vi "Dashboard Main.vi"() -> ()   [LabVIEW 2012]
uses:
  <vilib>/Rock Robotics/WPI/Solenoid/WPI_SolenoidValue.ctl
  <vilib>/event_ctls.llb/eventvkey.ctl
  <vilib>/Utility/config.llb/Read Key (String).vi
  <vilib>/Utility/config.llb/Read Key (I32).vi
  <vilib>/Utility/config.llb/Write Key (String).vi
  <vilib>/Utility/config.llb/Write Key (I32).vi
  <vilib>/Utility/config.llb/NI_LVConfig.lvlib
panel:
  in  "Run 2":bool
  in  "Run":bool
  in  "Far Speed":dbl=3850.0
  in  "Tower Speed":dbl=2500.0
  out "Camera Image 2":T1(plugin-control)
  in  "Time Delay":dbl
  out "Error":dbl(graph)
  in  "Listbox":i32(listbox)
  out "Shooter Angle":T2
  out "Climb Retical":bool
  out "Primary":T3 {"Slide" scale=-1.0..1.0; "Trigger" scale=-1.0..1.0}
  in  "stop? (T)":bool
  out "RPM":dbl(slide) scale=0.0..5000.0
  out "Right":dbl(slide) scale=-1.0..1.0
  out "Left":dbl(slide) scale=-1.0..1.0
  out "Battery Value":dbl(slide) scale=0.0..14.0 scale format="%#_2e"
  out "Battery":sgl(graph)
  in  "Camera Settings":T4={"Frate Rate"=30, "Compression"=30, "Size"=1} {"Frate Rate" scale=1.0..30.0; "Size" items=["640x480", "320x240", "160x120"]}
  out "Mode":T5(ring)=enum."Auto Disabled"
  out "Camera IP":string
  out "Robot IP":string
  in  "Dashboard Tab":enum32{"Operation", "Test", "Checklist"}(tab)
  in  "Slider":dbl(slide) scale=0.0..100.0 scale format="%#_3g"
  in  "On/Off":bool caption="Solenoid"
  in  "Test Name":u16(ring) items=["Select the test to run...", "Example Test", "-------------------------------", "List of tests is built in robot code.", "Replace with your own automated tests."]
  in  "Test Tree":string(tree)
  in  "Motor":cluster{"Value":dbl, "Enable":bool} {"Value" scale=-1.0..1.0 scale format="%#_3g"}
  out "Progress":T6 {"Test Progress" scale=0.0..100.0}
  in  "Rev/Fwd":cluster{"Forward":bool, "Reverse":bool}
  in  "Ring":u16(ring) items=["Auto", "Fixed indoor", "Fixed outdoor 1", "Fixed outdoor 2", "Fixed fluorescent 1", "Fixed fluorescent 2", "Hold current"]
  in  "Viewer":enum32{"Camera Image", "Variables"}(tab)
  out "Mbps":dbl format="%#.1g"
  in  "Enable":bool=TRUE
  in  "DB Camera Config":bool
  out "Mbps":bool
  out "fps":dbl format="%#.1g"
  out "Image Error Message":string="Timeout in Camera Communications"
  out "Tree":string(tree)
  # "Drive & Motors"
  # "Robot IP:"
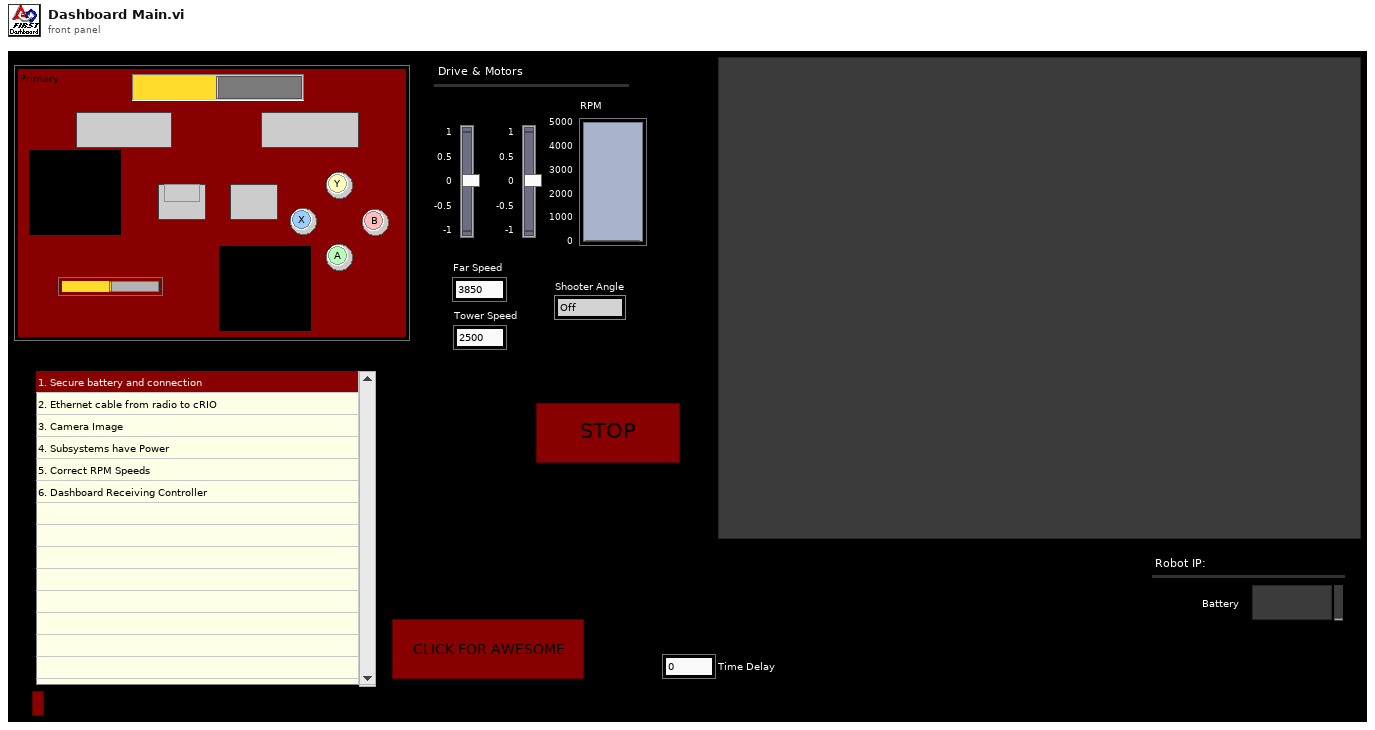
[diagram p1: front panel]
types:
  T1 = typedef "IMAQ Image.ctl" = refnum<image>
  T2 = typedef "WPI_SolenoidValue.ctl" = enum16{"Off", "On", "Forward", "Reverse"}
  T3 = cluster{"Y":bool, "B":bool, "X":bool, "A":bool, "Left Bumper":bool, "Right Bumper":bool, "Joystick 2":cluster{"X":dbl, "Y":dbl}[], "Joystick 3":cluster{"X":dbl, "Y":dbl}[], "Back":bool, "Start":bool, "Trigger":dbl, "Slide":dbl, "Right Thumbstick":bool, "Left Thumbstick":bool}
  T4 = cluster{"Frate Rate":i32, "Compression":i32, "Size":u16}
  T5 = enum8{"Tele-Op Disabled", "Tele-Op Enabled", "Auto Disabled", "Auto Enabled", "Test Disabled", "Test Enabled", ""}
  T6 = cluster{"Test Progress":u8, "Test Progress Text":string}
  T7 = typedef "Image Type" = u32
  T8 = typedef "LVRectTypeDef.ctl" = cluster{"Left":i16, "Top":i16, "Right":i16, "Bottom":i16}
  T9 = cluster{"Joy Stick":cluster{"Primary":cluster{"Buttons":cluster{"A":bool, "B":bool, "X":bool, "Y":bool, "Left Bumper":bool, "Right Bumper":bool, "Back":bool, "Start":bool, "Left Thumbstick":bool, "Right Thumbstick":bool}, "Axes":cluster{"Left Stick X ":dbl, "Left Stick Y":dbl, "Triggers":dbl, "Right Stick X":dbl, "Right Stick Y":dbl, "D-Pad X":dbl}}, "Secondary":cluster{"Buttons":cluster{"A":bool, "B":bool, "X":bool, "Y":bool, "Left Bumper":bool, "Right Bumper":bool, "Back":bool, "Start":bool, "Left Thumbstick":bool, "Right Thumbstick":bool}, "Axes":cluster{"Left Stick X ":dbl, "Left Stick Y":dbl, "Triggers":dbl, "Right Stick X":dbl, "Right Stick Y":dbl, "D-Pad X":dbl}}}, "Shooter":cluster{"RPM Current":dbl, "RPM Set":dbl, "In Range?":bool}, "Arm":cluster{"Arm Current":dbl, "Arm Set":dbl, "At Position?":bool, "Reset Encoder":bool}, "Drive":cluster{"Right":dbl, "Left":dbl}, "Climb State":enum16{"Arm Wait", "Arm Up", "Arm Down", "Arm Attach"}, "Change Retical":bool, "Solenoids":cluster{"Robot Angle":T2, "Shooter Angle":T2, "Arm Lock":T2}, "Shooter Speeds":dbl[]}
  T10 = cluster{"Competition mode":bool, "Robot Link":bool, "Autonomous":bool, "Enabled":bool, "E-Stop":bool, "Simulated":bool, "TestMode":bool, "Docked Window":bool}
  T11 = cluster{"Buttons":cluster{"A":bool, "B":bool, "X":bool, "Y":bool, "Left Bumper":bool, "Right Bumper":bool, "Back":bool, "Start":bool, "Left Thumbstick":bool, "Right Thumbstick":bool}, "Axes":cluster{"Left Stick X ":dbl, "Left Stick Y":dbl, "Triggers":dbl, "Right Stick X":dbl, "Right Stick Y":dbl, "D-Pad X":dbl}}
  T12 = typedef "NI_LVConfig.lvlib/Config Data RefNum.ctl" = refnum<k1>
  T13 = typedef "eventvkey.ctl" = enum16{"ASCII", "Enter", "Return", "Shift", "Ctrl", "Alt", "Cmd", "Opt", "Caps", "NumLock", "Clear", "Break", "Up", "Down", "Left", "Right", "Insert", "Delete", "Home", "End", "PageUp", "PageDown", "Escape", "Help", "Pause", "ScrollLock", "F1", "F2", "F3", "F4", "F5", "F6", "F7", "F8", "F9", "F10", "F11", "F12", "F13", "F14", "F15", "F16", "F17", "F18", "F19", "F20", "F21", "F22", "F23", "F24", "Play", "VolumeUp", "VolumeDown", "Mute", "Two Byte Char"}
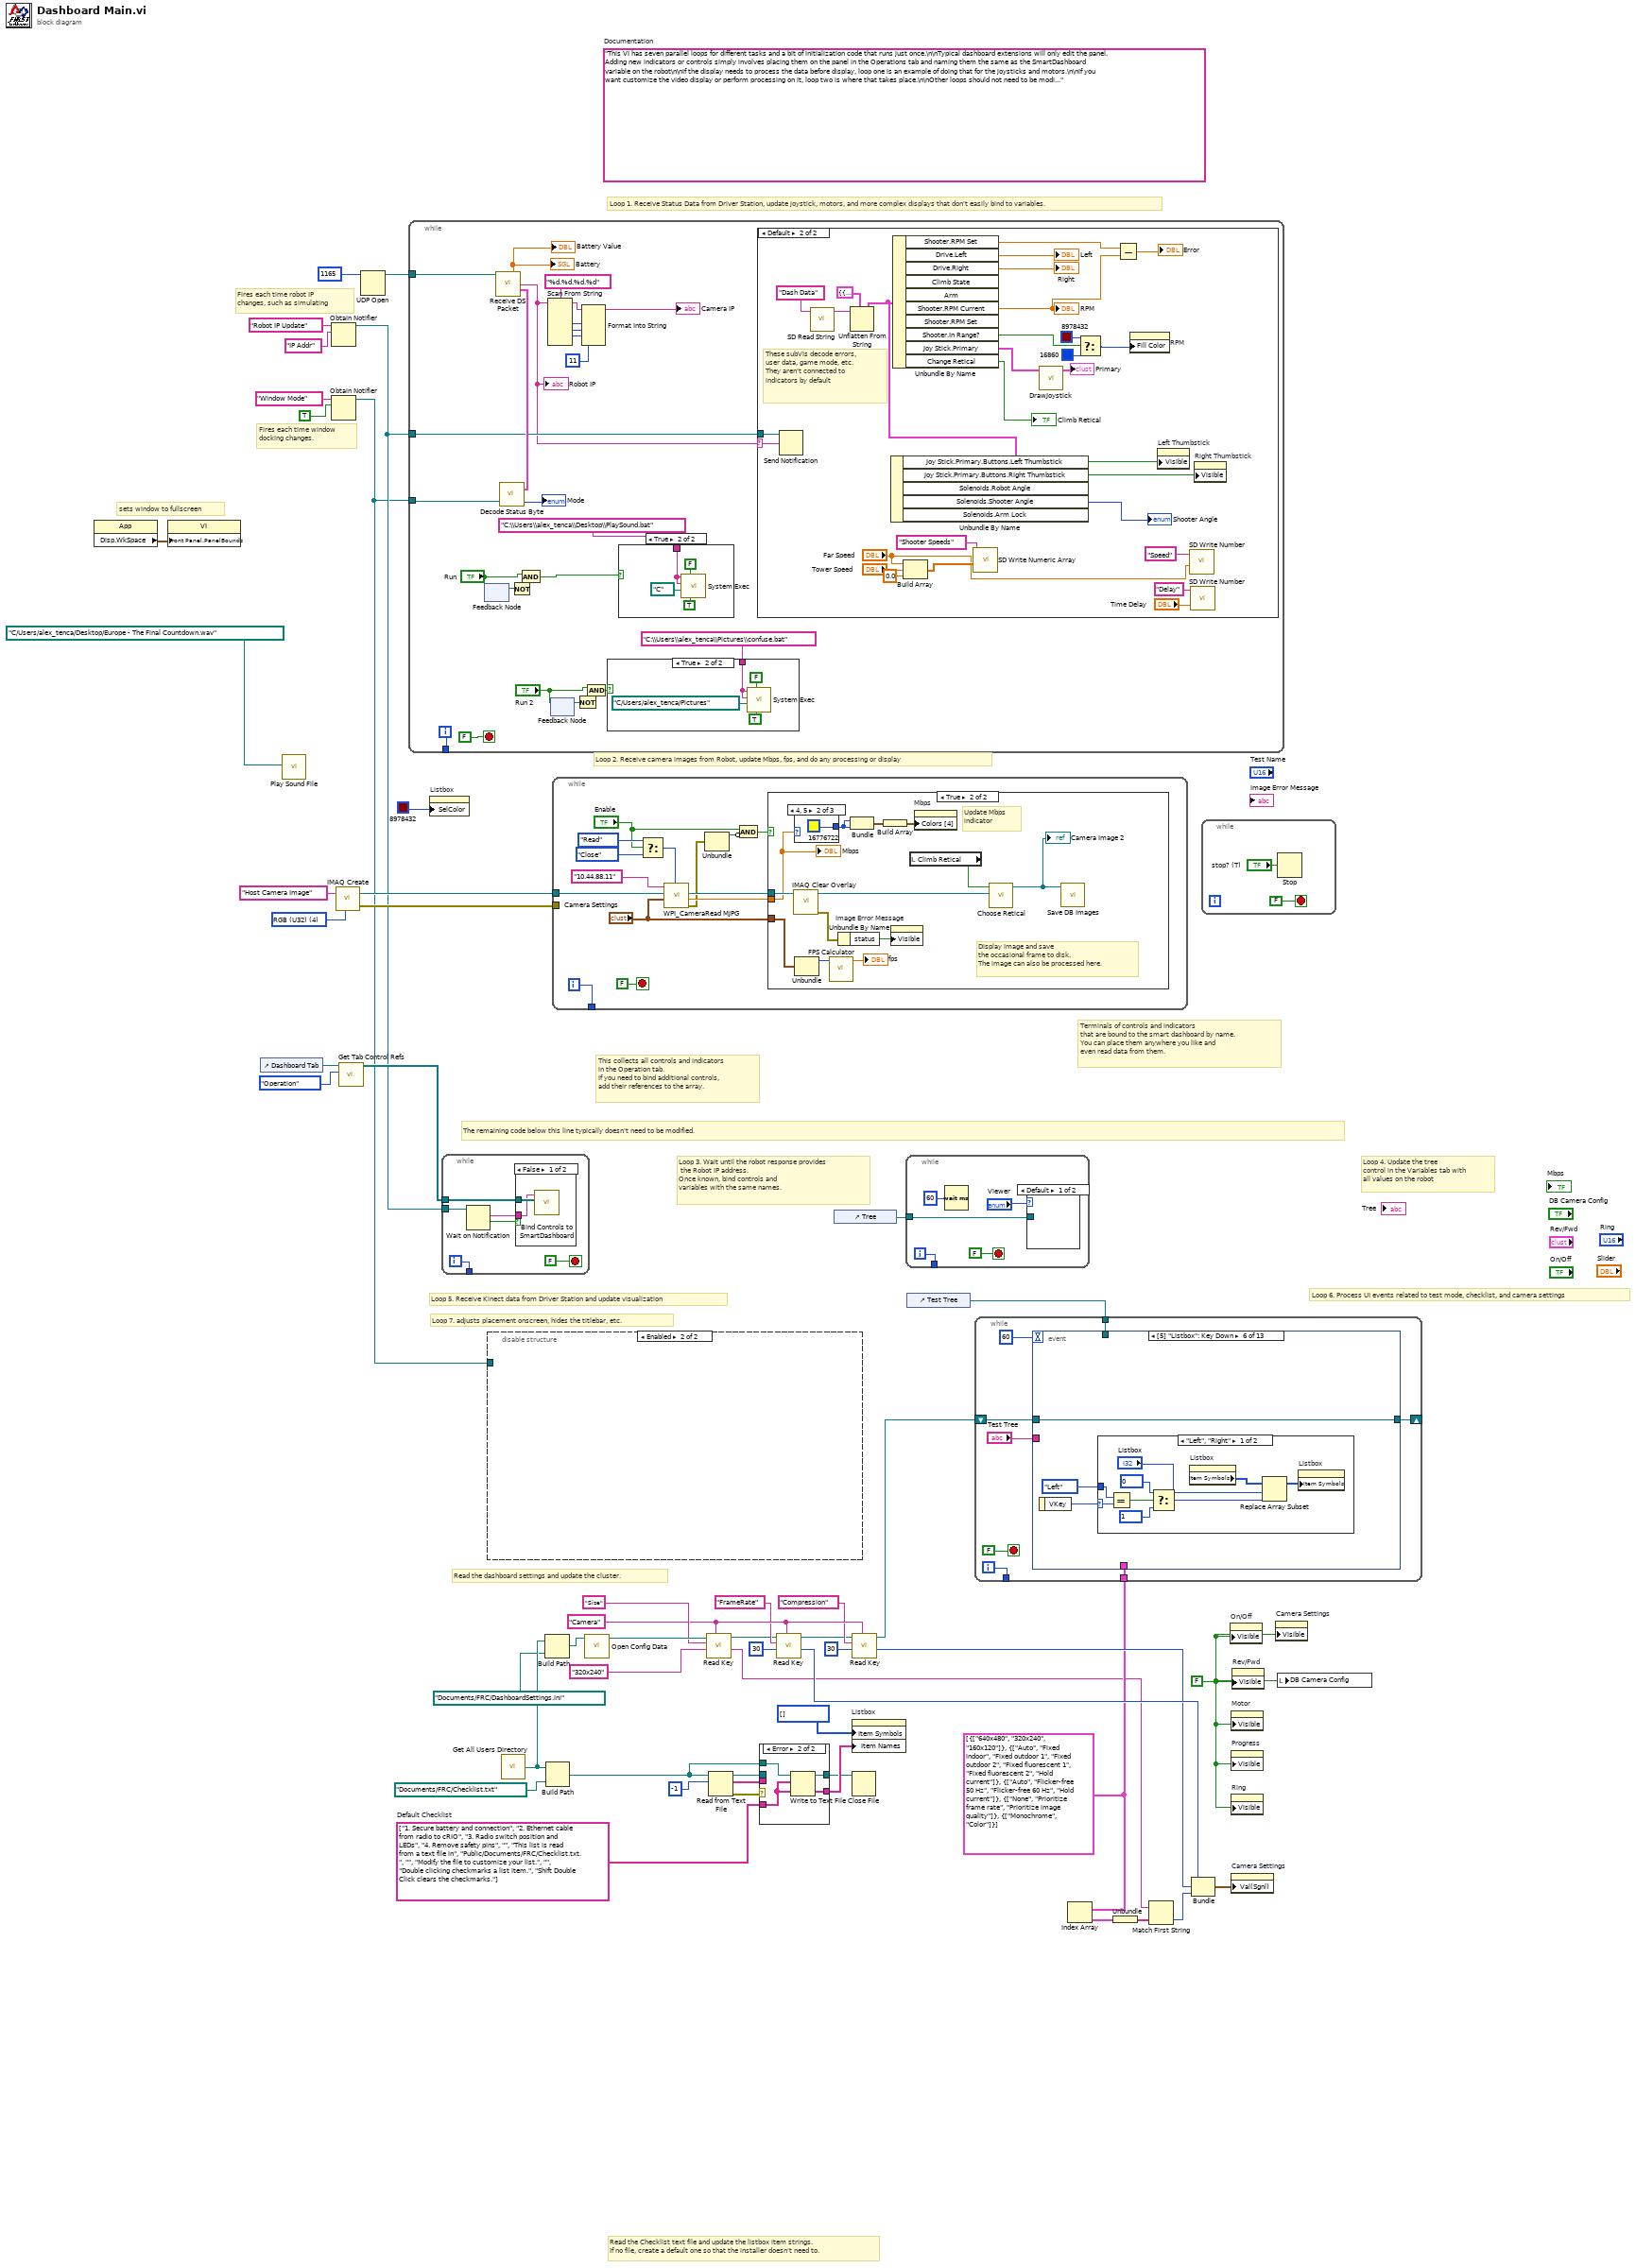
[diagram p0: block diagram]
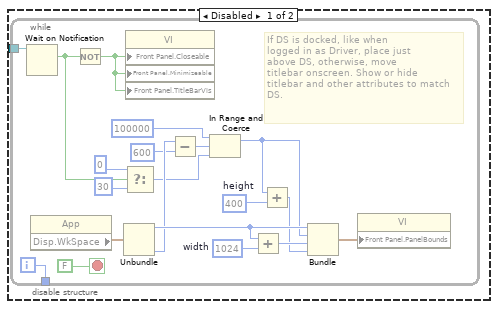
[diagram p2: hidden frame]
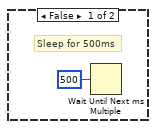
[diagram p4: hidden frame]
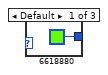
[diagram p5: hidden frame]
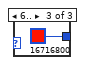
[diagram p6: hidden frame]
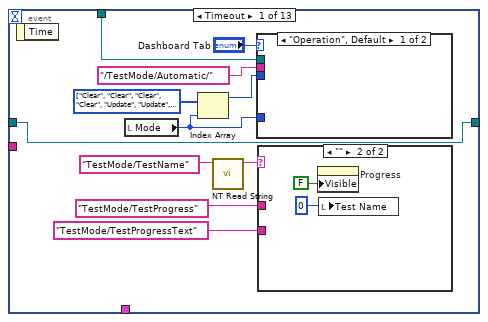
[diagram p8: hidden frame]
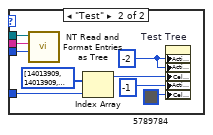
[diagram p9: hidden frame]
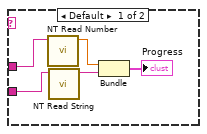
[diagram p10: hidden frame]
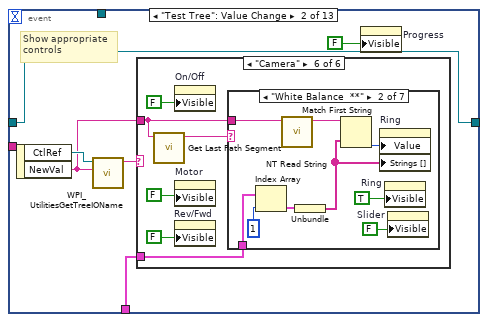
[diagram p11: hidden frame]
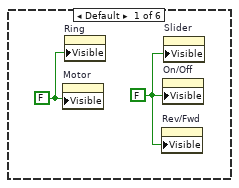
[diagram p12: hidden frame]
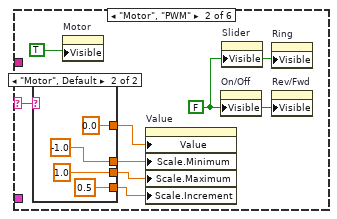
[diagram p13: hidden frame]
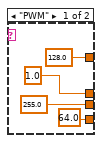
[diagram p14: hidden frame]
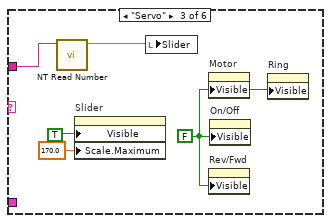
[diagram p15: hidden frame]
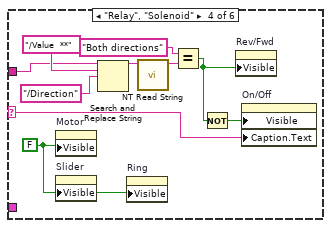
[diagram p16: hidden frame]
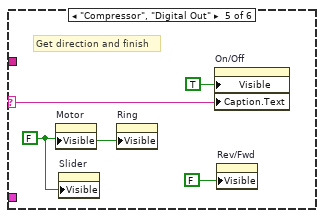
[diagram p17: hidden frame]
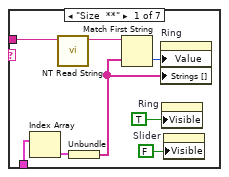
[diagram p18: hidden frame]
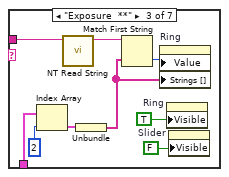
[diagram p19: hidden frame]
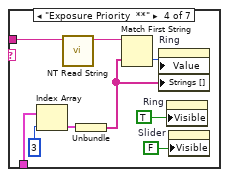
[diagram p20: hidden frame]
diagram:
  w25 = "Camera"
  w17 = cluster{string[]}[] [{["640x480", "320x240", "160x120"]}, {["Auto", "Fixed indoor", "Fixed outdoor 1", "Fixed outdoor 2", "Fixed fluorescent 1", "Fixed fluorescent 2", "Hold current"]}, {["Auto", "Flicker-free 50 Hz", "Flicker-free 60 Hz", "Hold current"]}, {["None", "Prioritize frame rate", "Prioritize image quality"]}, {["Monochrome", "Color"]}]
  w33 = string[] ["1. Secure battery and connection", "2. Ethernet cable from radio to cRIO", "3. Radio switch position and LEDs", "4. Remove safety pins", "", "This list is read from a text file in", "Public/Documents/FRC/Checklist.txt.", "", "Modify the file to customize your list.", "", "Double clicking checkmarks a list item.", "Shift Double Click clears the checkmarks."]  # Default Checklist
  w31 = FALSE ("Visible")
  (unwired) "This VI has seven parallel loops for different tasks and a bit of initialization code that runs just once.\n\nTypical dashboard extensions will only edit the panel. Adding new indicators or controls simply involves placing them on the panel in the Operations tab and naming them the same as the SmartDashboard variable on the robot\n\nIf the display needs to process the data before display, loop one is an example of doing that for the joysticks and motors.\n\nIf you want customize the video display or perform processing on it, loop two is where that takes place.\n\nOther loops should not need to be modified. They are pretty standard, and document the task they perform."  # Documentation
  w51 = T7 4 items=["Grayscale (U8)", "Grayscale (I16)", "Grayscale (SGL)", "Complex (CSG)", "RGB (U32)", "HSL (U32)", "RGB (U64)"] ("Image Type")
  # "sets window to fullscreen"
  # "Fires each time robot IP\nchanges, such as simulating"
  # "Fires each time window\ndocking changes."
  # "Read the Checklist text file and update the listbox item strings.\nIf no file, create a default one so that the installer doesn't need to."
  # "This collects all controls and indicators\nin the Operation tab.\nIf you need to bind additional controls,\nadd their references to the array."
  # "The remaining code below this line typically doesn't need to be modified."
  # "Loop 6. Process UI events related to test mode, checklist, and camera settings"
  # "Read the dashboard settings and update the cluster."
  # "Terminals of controls and indicators\nthat are bound to the smart dashboard by name.\nYou can place them anywhere you like and\neven read data from them."
  # "Loop 4. Update the tree\ncontrol in the Variables tab with\nall values on the robot"
  # "Loop 3. Wait until the robot response provides\n the Robot IP address.\nOnce known, bind controls and\nvariables with the same names."
  # "Loop 5. Receive Kinect data from Driver Station and update visualization"
  # "Loop 7. adjusts placement onscreen, hides the titlebar, etc."
  # "Loop 1. Receive Status Data from Driver Station, update joystick, motors, and more complex displays that don't easily bind to variables."
  # "Loop 2. Receive camera images from Robot, update Mbps, fps, and do any processing or display"
  n1 = property class="App"() -> ("Disp.WkSpace"=w4:T8)  [unwired: 2 in, 2 out]
  n2 = property class="VI"("Front Panel.PanelBounds"=w4) -> ()  [unwired: 2 in, 2 out]
  n3 = control-ref of="Dashboard Tab"() -> (w46:refnum<vi>)
  n4 = call <vilib>:"Play Sound File.vi"("path"=path "C:/Users/alex_tenca/Desktop/Europe - The Final Countdown.wav") -> ()  [unwired: 9 in, 2 out]
  n5 = Obtain Notifier(name (unnamed)="Robot IP Update", notification data type="IP Addr" ("name (unnamed)")) -> (notifier out=w43:refnum<notifier>)  [unwired: 2 in, 2 out]
  n6 = Obtain Notifier(name (unnamed)="Window Mode", notification data type=TRUE) -> (notifier out=w1:refnum<notifier>)  [unwired: 2 in, 2 out]
  n7 = call "IMAQ Create"("Image Name"="Host Camera Image", "Image Type"=w51) -> ("New Image"=w49:T1, "error out"=w48:errorcluster)  [unwired: 2 in, 1 out]
  n8 = call <vilib>:"Get Tab Control Refs.vi"("Page Index"=enum32{"Operation", "Test"}."Operation" ("Dashboard Tab"), "TabControl in"=w46) -> ("ControlsOnPage"=w47:refnum<vi>[])  [unwired: 9 in]
  n9 = UDP Open(11:u16 1165 ("port")) -> (port=w52:refnum<k16>)  [unwired: 2 in, 4 out]
  n10 = while {
    tunnel: w52 -> [w77]
    tunnel: w43 -> [w72]
    tunnel: w1 -> [w75]
    tunnel: [w73] -> _
    i -> [w73]
    stop <- FALSE stop-if-true
    n11 = feedback-in #1("Run") -> ()
    n12 = feedback #1() -> (w62:bool)  [unwired: 1 in]
    n13 = call "Receive DS Packet.vi"("Recv Socket"=w77) -> ("Battery"=→"Battery" →"Battery Value":sgl, "Robot IP Address"=w66:string, "Status"=w78:T10)  [unwired: 1 in, 11 out]
    "Robot IP" <- w66
    n14 = call "Decode Status Byte.vi"("Window Mode Notifier"=w75, "Status"=w78) -> ("Mode"=→"Mode":T5)  [unwired: 1 out]
    n15 = Not(x=w62) -> (.not. x?=w60:bool)
    n16 = And(x="Run", y=w60) -> (x .and. y?=w63:bool)
    n17 = Scan From String(format string="%d.%d.%d.%d", input string=w66) -> (remaining string=w64:string, output 1=w71:i32, output 2=w70:i32, output 3=w69:i32)  [unwired: 2 in, 7 out]
    n18 = feedback #2() -> (w57:bool)  [unwired: 1 in]
    n19 = feedback-in #2("Run 2") -> ()
    n20 = Not(x=w57) -> (.not. x?=w55:bool)
    n21 = Format Into String(initial string=w64, w71, w70, w69, 11 ("IP Suffix:")) -> (resulting string=→"Camera IP":string)  [unwired: 2 in, 1 out]
    n22 = And(x="Run 2", y=w55) -> (x .and. y?=w58:bool)
    n23 = case shown="True" w58 {
      tunnel: "C:\\Users\\alex_tenca\\Pictures\\confuse.bat" ("command line") -> [_ w80]
      frame False {
      }
      frame True {
        n24 = call <vilib>:"System Exec.vi"("run minimized? (F)"=TRUE, "wait until completion? (T)"=FALSE, "working directory"=path "C:/Users/alex_tenca/Pictures", "standard input"=w80, "command line"=w80) -> ()  [unwired: 3 in, 4 out]
      }
    }
    n25 = case shown="True" w63 {
      tunnel: "C:\\Users\\alex_tenca\\Desktop\\PlaySound.bat" ("command line") -> [_ w84]
      frame False {
      }
      frame True {
        n26 = call <vilib>:"System Exec.vi"("run minimized? (F)"=TRUE, "wait until completion? (T)"=FALSE, "working directory"=path "C:/", "standard input"=w84, "command line"=w84) -> ()  [unwired: 3 in, 4 out]
      }
    }
    n27 = case shown="Default" w66 {
      selector: w66 -> [_ w115]
      tunnel: w72 -> [_ w116]
      frame "0.0.0.0" {
        # "Robot not responding, don't poll the variables"
      }
      frame Default {
        # "These subVIs decode errors, user data, game mode, etc.\nThey aren't connected to indicators by default"
        n28 = Send Notification(notification=w115, notifier=w116) -> ()  [unwired: 1 in, 2 out]
        n29 = call <vilib>:"SD Read String.vi"("Name"="Dash Data") -> ("String"=w113:string)  [unwired: 8 in, 2 out]
        n30 = Unflatten From String(type=T9 {"Joy Stick"={"Primary"={"Buttons"={"A"=FALSE, "B"=FALSE, "X"=FALSE, "Y"=FALSE, "Left Bumper"=FALSE, "Right Bumper"=FALSE, "Back"=FALSE, "Start"=FALSE, "Left Thumbstick"=FALSE, "Right Thumbstick"=FALSE}, "Axes"={"Left Stick X "=0.0, "Left Stick Y"=0.0, "Triggers"=-0.0, "Right Stick X"=0.0, "Right Stick Y"=0.0, "D-Pad X"=0.0}}, "Secondary"={"Buttons"={"A"=FALSE, "B"=FALSE, "X"=FALSE, "Y"=FALSE, "Left Bumper"=FALSE, "Right Bumper"=FALSE, "Back"=FALSE, "Start"=FALSE, "Left Thumbstick"=FALSE, "Right Thumbstick"=FALSE}, "Axes"={"Left Stick X "=0.0, "Left Stick Y"=0.0, "Triggers"=0.0, "Right Stick X"=0.0, "Right Stick Y"=0.0, "D-Pad X"=0.0}}}, "Shooter"={"RPM Current"=0.0, "RPM Set"=0.0, "In Range?"=FALSE}, "Arm"={"Arm Current"=0.0, "Arm Set"=0.0, "At Position?"=FALSE, "Reset Encoder"=FALSE}, "Drive"={"Right"=0.0, "Left"=0.0}, "Climb State"=enum."Arm Attach", "Change Retical"=FALSE, "Solenoids"={"Robot Angle"=enum."Off", "Shooter Angle"=enum."Off", "Arm Lock"=enum."Off"}, "Shooter Speeds"=[0.0, 0.0, 0.0]} ("Dash Data"), binary string=w113) -> (value=w109:T9)  [unwired: 3 in, 2 out]
        n31 = Unbundle By Name(w109) -> ("Joy Stick.Primary.Buttons.Left Thumbstick"=w99:bool, "Joy Stick.Primary.Buttons.Right Thumbstick"=w98:bool, "Solenoids.Shooter Angle"=→"Shooter Angle":T2)  [unwired: 2 out]
        n32 = Unbundle By Name(w109) -> ("Shooter.RPM Set"=w107:dbl, "Drive.Left"=→"Left":dbl, "Drive.Right"=→"Right":dbl, "Shooter.RPM Current"=w106:dbl, "Shooter.In Range?"=w104:bool, "Joy Stick.Primary"=w110:T11, "Change Retical"=→"Climb Retical":bool)  [unwired: 3 out]
        "RPM" <- w106
        n33 = Build Array("Far Speed", "Tower Speed", 0.0 ("element")) -> (w92:dbl[])
        n34 = call <vilib>:"SD Write Numeric Array.vi"("Numeric Array"=w92, "Name"="Shooter Speeds") -> ()  [unwired: 8 in, 2 out]
        n35 = call "DrawJoystick.vi"("Joystick"=w110) -> ("DrawJoy"=→"Primary":T3)  [unwired: 10 in]
        n36 = Select(t=u32 8978432 ("Color Box"), s=w104, f=u32 16860 ("Color Box")) -> (s? t:f=w102:u32)
        n37 = Subtract(x=w107, y=w106) -> (x-y=→"Error":dbl)
        n38 = property on="RPM" class="Slide (strict)"("Fill Color"=w102) -> ()  [unwired: 2 in, 2 out]
        n39 = property on="Left Thumbstick" class="Bool (strict)"("Visible"=w99) -> ()  [unwired: 2 in, 2 out]
        n40 = call <vilib>:"SD Write Number.vi"("Numeric"="Far Speed", "Name"="Speed") -> ()  [unwired: 8 in, 2 out]
        n41 = call <vilib>:"SD Write Number.vi"("Numeric"="Time Delay", "Name"="Delay") -> ()  [unwired: 8 in, 2 out]
        n42 = property on="Right Thumbstick" class="Bool (strict)"("Visible"=w98) -> ()  [unwired: 2 in, 2 out]
      }
    }
  }
  n43 = property on="Listbox" class="LstBox (strict)"("SelColor"=u32 8978432 ("Color Box")) -> ()  [unwired: 2 in, 2 out]
  n44 = while {
    tunnel: w47 -> [w122]
    tunnel: w43 -> [w119]
    tunnel: [w117] -> _
    i -> [w117]
    stop <- FALSE stop-if-true
    n45 = Wait on Notification(notifier=w119) -> (notification=w118:string, timed out?=w120:bool)  [unwired: 3 in, 2 out]
    n46 = case shown="False" w120 {
      tunnel: w122 -> [w124 _]
      tunnel: w118 -> [w123 _]
      frame False {
        n47 = call <vilib>:"Bind Controls to SmartDashboard.vi"("Bound Control Refs"=w124, "Server IP Address"=w123) -> ()  [unwired: 10 in]
      }
      frame True {
      }
    }
  }
  n48 = disable-structure shown="Enabled" {
    disable-tunnel: w1 -> [w125 _]
    frame Disabled {
      n49 = while {
        tunnel: w125 -> [w144]
        tunnel: [w142] -> _
        i -> [w142]
        stop <- FALSE stop-if-true
        w134 = 1024  # width
        w137 = 400  # height
        # "If DS is docked, like when\nlogged in as Driver, place just\nabove DS, otherwise, move\ntitlebar onscreen. Show or hide\ntitlebar and other attributes to match\nDS."
        n50 = Wait on Notification(notifier=w144) -> (notification=w129:bool)  [unwired: 3 in, 3 out]
        n51 = property class="App"() -> ("Disp.WkSpace"=w140:T8)  [unwired: 2 in, 2 out]
        n52 = Not(x=w129) -> (.not. x?=w143:bool)
        n53 = Unbundle(w140) -> ("Left"=w138:i16, "Bottom"=w135:i16)  [unwired: 2 out]
        n54 = Select(t=0, s=w129, f=30) -> (s? t:f=w128:i32)
        n55 = property class="VI"("Front Panel.Closeable"=w143, "Front Panel.Minimizeable"=w143, "Front Panel.TitleBarVis"=w143) -> ()  [unwired: 2 in, 2 out]
        n56 = Subtract(x=w135, y=600) -> (x-y=w132:i32)
        n57 = In Range and Coerce(upper limit=100000, x=w132, lower limit=w128) -> (coerced(x)=w126:i32)  [unwired: 1 out]
        n58 = Add(x=w138, y=w134) -> (x+y=w139:i32)
        n59 = Add(x=w126, y=w137) -> (x+y=w136:i32)
        n60 = Bundle("Left"=w138, w126, w139, w136) -> (w141:cluster{"Left":i16, i32, i32, i32})  [unwired: 1 out]
        n61 = property class="VI"("Front Panel.PanelBounds"=w141) -> ()  [unwired: 2 in, 2 out]
      }
    }
    frame Enabled {
    }
  }
  n62 = call "Get All Users Directory.vi"() -> ("All User Path"=w30:path)
  n63 = Build Path(base path=w30, name or relative path=path "Documents/FRC/DashboardSettings.ini") -> (appended path=w29:path)
  n64 = Build Path(base path=w30, name or relative path=path "Documents/FRC/Checklist.txt") -> (appended path=w34:path)
  n65 = while {
    tunnel: w49 -> [w156]
    tunnel: w48 -> [_]
    tunnel: [w158] -> _
    i -> [w158]
    stop <- FALSE stop-if-true
    n66 = Select(t=enum16{"Read", "Reopen", "Close"}."Read" ("Operation"), s="Enable", f=enum16{"Read", "Reopen", "Close"}."Close" ("Operation")) -> (s? t:f=w151:enum16{"Read", "Reopen", "Close"})
    n67 = call <vilib>:"WPI_CameraRead MJPG.vi"("Operation"=w151, "Camera Settings"="Camera Settings", "Image"=w156, "address"="10.44.88.11") -> ("error out"=w150:errorcluster, "Bandwidth (kbps)"=w154:dbl, "Image Out"=w155:T1)  [unwired: 5 in]
    n68 = Unbundle(w150) -> ("status"=w148:bool)  [unwired: 2 out]
    n69 = Compound Arithmetic op=AND("Enable", invert w148) -> (w147:bool)
    n70 = case shown="True" w147 {
      tunnel: "Camera Settings" -> [_ w165]
      tunnel: w155 -> [_ w168]
      tunnel: w154 -> [_ w167]
      frame False {
        # "Sleep for 500ms"
        n71 = Wait Until Next ms Multiple(millisecond multiple=u32 500) -> ()  [unwired: 1 out]
      }
      frame True {
        # "Display image and save\nthe occasional frame to disk.\nThe image can also be processed here."
        # "Update Mbps\nindicator"
        n72 = call "IMAQ Clear Overlay"("Image"=w168) -> ("error out"=w172:errorcluster, "Image Out"=w162:T1)  [unwired: 2 in, 7 out]
        n73 = case shown="4, 5" w167 {
          tunnel: [u32 6618880 ("Color Box") u32 16776722 ("Color Box") u32 16716800 ("Color Box")] -> w169
          frame Default {
          }
          frame 4, 5 {
          }
          frame 6.. {
          }
        }
        n74 = Unbundle(w165) -> ("Frate Rate"=w164:i32)  [unwired: 2 out]
        n75 = call "FPS Calculator.vi"("Average Count"=w164) -> ("fps"=→"fps":dbl)  [unwired: 10 in]
        n76 = Unbundle By Name(w172) -> ("status"=w173:bool)
        n77 = Bundle("Color Box"=w169, "Color Box"=w169) -> (w171:cluster{"Color Box":u32, "Color Box":u32})  [unwired: 1 out]
        n78 = Build Array(w171) -> (w170:cluster{"Color Box":u32, "Color Box":u32}[])
        n79 = property on="Image Error Message" class="Str"("Visible"=w173) -> ()  [unwired: 2 in, 2 out]
        n80 = local read "Climb Retical"() -> (w163:bool)
        n81 = property on="Mbps" class="Bool (strict)"("Colors [4]"=w170) -> ()  [unwired: 2 in, 2 out]
        n82 = call "Choose Retical.vi"("Image In"=w162, "Climb Retical"=w163) -> ("Image Out"=w161:T1)  [unwired: 9 in]
        "Camera Image 2" <- w161
        n83 = call "Save DB Images.vi"("Image"=w161) -> ()  [unwired: 2 in, 1 out]
        "Mbps" <- w167
      }
    }
  }
  n84 = call <vilib>:"Open Config Data.vi"("configuration file path"=w29) -> ("refnum"=w28:T12)  [unwired: 8 in, 2 out]
  n85 = call-poly <vilib>:"Read Key.vi"("section"=w25, "default value"="320x240", "key"="Size", "refnum"=w28) -> ("value"=w15:string, "refnum out"=w10:T12)  [unwired: 2 in, 4 out]
  n86 = Read from Text File(file (use dialog)=w34, count=-1 ("timeout ms (25000)")) -> (refnum out=w12:refnum<file>, text=w35:string[], error out=w36:errorcluster)  [unwired: 2 in, 1 out]
  n87 = case shown="Error" w36 {
    tunnel: w35 -> [w178 _]
    tunnel: [w178 w180] -> w32
    tunnel: w33 -> [_ w180]
    tunnel: w34 -> [_ w181]
    tunnel: [w177 w179] -> w11
    tunnel: w12 -> [w177 _]
    frame No Error {
    }
    frame Error {
      n88 = Write to Text File(file (use dialog)=w181, text=w180) -> (refnum out=w179:refnum<file>)  [unwired: 2 in, 2 out]
    }
  }
  n89 = call-poly <vilib>:"Read Key.vi"("section"=w25, "default value"=30, "key"="FrameRate", "refnum"=w10) -> ("value"=w20:i32, "refnum out"=w9:T12)  [unwired: 1 in, 5 out]
  n90 = control-ref of="Tree"() -> (w6:refnum<vi>)
  n91 = property on="Listbox" class="LstBox (strict)"("Item Symbols"=i32[] [], "Item Names"=w32) -> ()  [unwired: 2 in, 2 out]
  n92 = Close File(refnum=w11) -> ()  [unwired: 1 in, 2 out]
  n93 = call-poly <vilib>:"Read Key.vi"("section"=w25, "default value"=30, "key"="Compression", "refnum"=w9) -> ("value"=w19:i32, "refnum out"=w7:T12)  [unwired: 1 in, 5 out]
  n94 = while {
    tunnel: [w183] -> _
    tunnel: w6 -> [w182]
    i -> [w183]
    stop <- FALSE stop-if-true
    n95 = Wait (ms)(milliseconds to wait=u32 60) -> ()  [unwired: 1 out]
    n96 = case shown="Default" "Viewer" {
      tunnel: w182 -> [_ w187]
      frame Default {
      }
      frame "Variables" {
        n97 = call <vilib>:"NT Read and Format Entries as Tree.vi"("Tree Refnum"=w187) -> ()  [unwired: 9 in, 2 out]
      }
    }
  }
  n98 = control-ref of="Test Tree"() -> (w5:refnum<vi>)
  n99 = while {
    tunnel: w17 -> [w192]
    shift-right: [w191] -> _
    shift-left: w7 -> [w190]
    tunnel: [w189] -> _
    tunnel: w5 -> [w188]
    i -> [w189]
    stop <- FALSE stop-if-true
    n100 = event shown="[5] \"Listbox\": Key Down" {
      selector: _ -> [_ _ _ _ _ _ _ _ _ _ _ _ _]
      dyn-events: _ -> [_ _ _ _ _ _ _ _ _ _ _ _ _]
      timeout: u32 60 ("milliseconds to wait") -> [_ _ _ _ _ _ _ _ _ _ _ _ _]
      tunnel: w188 -> [w202 _ _ _ _ _ _ _ _ _ _ _ _]
      tunnel: "Test Tree" -> [_ _ _ _ _ _ _ _ w396 w404 w406 w410 w418]
      tunnel: w192 -> [_ w224 _ _ _ _ w360 w390 _ _ _ _ _]
      tunnel: [w196 w223 _ w326 w334 w346 w359 w383 w395 w402 w405 w409 w417] -> w191
      tunnel: w190 -> [w196 w223 _ w326 w334 w346 w358 w383 w395 w402 w405 w409 w417]
      event Timeout {
        w201 = enum16{"Update", "Clear"}[] [enum."Clear", enum."Clear", enum."Clear", enum."Clear", enum."Update", enum."Update", enum."Clear"] items=["Update", "Clear"]
        n101 = event-data() -> ()  [unwired: 1 in, 1 out]
        n102 = local read "Mode"() -> (w199:T5)
        n103 = Index Array(array=w201, index=w199) -> (element=w200:enum16{"Update", "Clear"})
        n104 = call <vilib>:"NT Read String.vi"("Name"="TestMode/TestName") -> ("String"=w205:string)  [unwired: 9 in, 1 out]
        n105 = case shown="\"Operation\", Default" "Dashboard Tab" {
          tunnel: w202 -> [_ w215]
          tunnel: "/TestMode/Automatic/" ("Name Pattern") -> [_ w214]
          tunnel: w200 -> [_ w213]
          tunnel: w199 -> [_ w211]
          frame "Operation", Default {
          }
          frame "Test" {
            w210 = -2 ("Active Item:Row Number")
            n106 = call <vilib>:"NT Read and Format Entries as Tree.vi"("Operation"=w213, "Name Pattern"=w214, "Tree Refnum"=w215) -> ()  [unwired: 7 in, 2 out]
            n107 = Index Array(array=u32[] [14013909, 14013909, 14013909, 14013909, 14013909, 16777215, 14013909], index=w211) -> (element=w209:u32)
            n108 = property on="Test Tree" class="Tree (strict)"("Active Item Row Number"=w210, "ActiveColNum"=w210, "CellBG"=w209, "Active Item Row Number"=-1 ("Active Item:Row Number"), "CellBG"=u32 5789784 ("Color Box")) -> ()  [unwired: 2 in, 2 out]
          }
        }
        n109 = case shown="\"\"" w205 {
          tunnel: "TestMode/TestProgress" ("Name") -> [w217 _]
          tunnel: "TestMode/TestProgressText" ("Name") -> [w216 _]
          frame Default {
            n110 = call <vilib>:"NT Read Number.vi"("Name"=w217) -> ("Numeric"=w218:dbl)  [unwired: 9 in, 1 out]
            n111 = call <vilib>:"NT Read String.vi"("Name"=w216) -> ("String"=w219:string)  [unwired: 9 in, 1 out]
            n112 = Bundle("Numeric"=w218, "String"=w219) -> (→"Progress":cluster{"Numeric":dbl, "String":string})  [unwired: 1 in]
          }
          frame "" {
            n113 = property on="Progress" class="Clust (strict)"("Visible"=FALSE) -> ()  [unwired: 2 in, 2 out]
            n114 = local write "Test Name"(u16 0) -> ()
          }
        }
      }
      event "Test Tree": Value Change {
        # "Show appropriate\ncontrols"
        n115 = event-data() -> ("CtlRef"=w227:refnum<vi>, "NewVal"=w225:string)  [unwired: 1 in]
        n116 = call <vilib>:"WPI_UtilitiesGetTreeIOName.vi"("NewVal"=w225, "TreeControl in"=w227) -> ("I/O Name"=w228:string)  [unwired: 9 in]
        n117 = case shown="\"Camera\"" w228 {
          selector: w228 -> [_ w235 _ w253 w262 _]
          tunnel: w225 -> [_ _ w250 w252 _ w269]
          tunnel: w224 -> [_ _ _ _ _ w268]
          frame Default {
            w230 = FALSE ("Visible")
            w229 = FALSE ("Visible")
            n118 = property on="Motor" class="Clust (strict)"("Visible"=w229) -> ()  [unwired: 2 in, 2 out]
            n119 = property on="Ring" class="Ring (strict)"("Visible"=w229) -> ()  [unwired: 2 in, 2 out]
            n120 = property on="Rev/Fwd" class="Clust (strict)"("Visible"=w230) -> ()  [unwired: 2 in, 2 out]
            n121 = property on="On/Off" class="Bool (strict)"("Visible"=w230) -> ()  [unwired: 2 in, 2 out]
            n122 = property on="Slider" class="Slide (strict)"("Visible"=w230) -> ()  [unwired: 2 in, 2 out]
          }
          frame "Motor", "PWM" {
            w236 = FALSE ("Visible")
            n123 = case shown="\"Motor\", Default" w235 {
              tunnel: [1.0 ("Value") -1.0 ("Value")] -> w234
              tunnel: [255.0 ("Value") 1.0 ("Value")] -> w233
              tunnel: [128.0 ("Value") 0.0 ("Value")] -> w232
              tunnel: [64.0 ("Value") 0.5 ("Value")] -> w231
              frame "PWM" {
              }
              frame "Motor", Default {
              }
            }
            n124 = property on="Motor" class="Clust (strict)"("Visible"=TRUE) -> ()  [unwired: 2 in, 2 out]
            n125 = property on="Value" class="Slide (strict)"("Value"=w232, "Scale.Minimum"=w234, "Scale.Maximum"=w233, "Scale.Increment"=w231) -> ()  [unwired: 2 in, 2 out]
            n126 = property on="On/Off" class="Bool (strict)"("Visible"=w236) -> ()  [unwired: 2 in, 2 out]
            n127 = property on="Slider" class="Slide (strict)"("Visible"=w236) -> ()  [unwired: 2 in, 2 out]
            n128 = property on="Ring" class="Ring (strict)"("Visible"=w236) -> ()  [unwired: 2 in, 2 out]
            n129 = property on="Rev/Fwd" class="Clust (strict)"("Visible"=w236) -> ()  [unwired: 2 in, 2 out]
          }
          frame "Servo" {
            w248 = FALSE ("Visible")
            n130 = call <vilib>:"NT Read Number.vi"("Name"=w250) -> ("Numeric"=w249:dbl)  [unwired: 9 in, 1 out]
            n131 = property on="Slider" class="Slide (strict)"("Visible"=TRUE, "Scale.Maximum"=170.0 ("Scale.Range:Maximum")) -> ()  [unwired: 2 in, 2 out]
            n132 = local write "Slider"(w249) -> ()
            n133 = property on="Motor" class="Clust (strict)"("Visible"=w248) -> ()  [unwired: 2 in, 2 out]
            n134 = property on="Rev/Fwd" class="Clust (strict)"("Visible"=w248) -> ()  [unwired: 2 in, 2 out]
            n135 = property on="On/Off" class="Bool (strict)"("Visible"=w248) -> ()  [unwired: 2 in, 2 out]
            n136 = property on="Ring" class="Ring (strict)"("Visible"=w248) -> ()  [unwired: 2 in, 2 out]
          }
          frame "Relay", "Solenoid" {
            w251 = FALSE ("Visible")
            n137 = property on="Motor" class="Clust (strict)"("Visible"=w251) -> ()  [unwired: 2 in, 2 out]
            n138 = property on="Slider" class="Slide (strict)"("Visible"=w251) -> ()  [unwired: 2 in, 2 out]
            n139 = Search and Replace String(input string=w252, search string="/Value  **", replace string="/Direction") -> (result string=w258:string)  [unwired: 5 in, 3 out]
            n140 = property on="Ring" class="Ring (strict)"("Visible"=w251) -> ()  [unwired: 2 in, 2 out]
            n141 = call <vilib>:"NT Read String.vi"("Name"=w258) -> ("String"=w256:string)  [unwired: 9 in, 1 out]
            n142 = Equal?(x="Both directions", y=w256) -> (x = y?=w254:bool)
            n143 = Not(x=w254) -> (.not. x?=w255:bool)
            n144 = property on="Rev/Fwd" class="Clust (strict)"("Visible"=w254) -> ()  [unwired: 2 in, 2 out]
            n145 = property on="On/Off" class="Bool (strict)"("Visible"=w255, "Caption.Text"=w253) -> ()  [unwired: 2 in, 2 out]
          }
          frame "Compressor", "Digital Out" {
            w261 = FALSE ("Visible")
            # "Get direction and finish"
            n146 = property on="Motor" class="Clust (strict)"("Visible"=w261) -> ()  [unwired: 2 in, 2 out]
            n147 = property on="Slider" class="Slide (strict)"("Visible"=w261) -> ()  [unwired: 2 in, 2 out]
            n148 = property on="Ring" class="Ring (strict)"("Visible"=w261) -> ()  [unwired: 2 in, 2 out]
            n149 = property on="On/Off" class="Bool (strict)"("Visible"=TRUE, "Caption.Text"=w262) -> ()  [unwired: 2 in, 2 out]
            n150 = property on="Rev/Fwd" class="Clust (strict)"("Visible"=FALSE) -> ()  [unwired: 2 in, 2 out]
          }
          frame "Camera" {
            n151 = call <vilib>:"Get Last Path Segment.vi"("String in"=w269) -> ("String out"=w270:string)  [unwired: 10 in]
            n152 = property on="On/Off" class="Bool (strict)"("Visible"=FALSE) -> ()  [unwired: 2 in, 2 out]
            n153 = property on="Motor" class="Clust (strict)"("Visible"=FALSE) -> ()  [unwired: 2 in, 2 out]
            n154 = property on="Rev/Fwd" class="Clust (strict)"("Visible"=FALSE) -> ()  [unwired: 2 in, 2 out]
            n155 = case shown="\"White Balance  **\"" w270 {
              tunnel: w269 -> [w276 w285 w294 w303 w312 _ w318]
              tunnel: w268 -> [w274 w282 w291 w300 w309 _ _]
              frame "Size  **" {
                n156 = Index Array(array=w274) -> (element=w273:cluster{string[]})  [unwired: 1 in]
                n157 = call <vilib>:"NT Read String.vi"("Name"=w276) -> ("String"=w275:string)  [unwired: 9 in, 1 out]
                n158 = Unbundle(w273) -> (w271:string[])
                n159 = Match First String(2:w271, 3:w275) -> (0:w272:i32)  [unwired: 1 out]
                n160 = property on="Ring" class="Ring (strict)"("Value"=w272, "Strings []"=w271) -> ()  [unwired: 2 in, 2 out]
                n161 = property on="Ring" class="Ring (strict)"("Visible"=TRUE) -> ()  [unwired: 2 in, 2 out]
                n162 = property on="Slider" class="Slide (strict)"("Visible"=FALSE) -> ()  [unwired: 2 in, 2 out]
              }
              frame "White Balance  **" {
                n163 = Index Array(array=w282, index=1) -> (element=w283:cluster{string[]})
                n164 = call <vilib>:"NT Read String.vi"("Name"=w285) -> ("String"=w284:string)  [unwired: 9 in, 1 out]
                n165 = Unbundle(w283) -> (w280:string[])
                n166 = Match First String(2:w280, 3:w284) -> (0:w279:i32)  [unwired: 1 out]
                n167 = property on="Ring" class="Ring (strict)"("Value"=w279, "Strings []"=w280) -> ()  [unwired: 2 in, 2 out]
                n168 = property on="Ring" class="Ring (strict)"("Visible"=TRUE) -> ()  [unwired: 2 in, 2 out]
                n169 = property on="Slider" class="Slide (strict)"("Visible"=FALSE) -> ()  [unwired: 2 in, 2 out]
              }
              frame "Exposure  **" {
                n170 = Index Array(array=w291, index=2) -> (element=w292:cluster{string[]})
                n171 = call <vilib>:"NT Read String.vi"("Name"=w294) -> ("String"=w293:string)  [unwired: 9 in, 1 out]
                n172 = Unbundle(w292) -> (w288:string[])
                n173 = Match First String(2:w288, 3:w293) -> (0:w289:i32)  [unwired: 1 out]
                n174 = property on="Ring" class="Ring (strict)"("Value"=w289, "Strings []"=w288) -> ()  [unwired: 2 in, 2 out]
                n175 = property on="Ring" class="Ring (strict)"("Visible"=TRUE) -> ()  [unwired: 2 in, 2 out]
                n176 = property on="Slider" class="Slide (strict)"("Visible"=FALSE) -> ()  [unwired: 2 in, 2 out]
              }
              frame "Exposure Priority  **" {
                n177 = Index Array(array=w300, index=3) -> (element=w301:cluster{string[]})
                n178 = call <vilib>:"NT Read String.vi"("Name"=w303) -> ("String"=w302:string)  [unwired: 9 in, 1 out]
                n179 = Unbundle(w301) -> (w297:string[])
                n180 = Match First String(2:w297, 3:w302) -> (0:w298:i32)  [unwired: 1 out]
                n181 = property on="Ring" class="Ring (strict)"("Value"=w298, "Strings []"=w297) -> ()  [unwired: 2 in, 2 out]
                n182 = property on="Ring" class="Ring (strict)"("Visible"=TRUE) -> ()  [unwired: 2 in, 2 out]
                n183 = property on="Slider" class="Slide (strict)"("Visible"=FALSE) -> ()  [unwired: 2 in, 2 out]
              }
              frame "Color Enable  **" {
                n184 = Index Array(array=w309, index=4) -> (element=w310:cluster{string[]})
                n185 = call <vilib>:"NT Read String.vi"("Name"=w312) -> ("String"=w311:string)  [unwired: 9 in, 1 out]
                n186 = Unbundle(w310) -> (w306:string[])
                n187 = Match First String(2:w306, 3:w311) -> (0:w307:i32)  [unwired: 1 out]
                n188 = property on="Ring" class="Ring (strict)"("Value"=w307, "Strings []"=w306) -> ()  [unwired: 2 in, 2 out]
                n189 = property on="Ring" class="Ring (strict)"("Visible"=TRUE) -> ()  [unwired: 2 in, 2 out]
                n190 = property on="Slider" class="Slide (strict)"("Visible"=FALSE) -> ()  [unwired: 2 in, 2 out]
              }
              frame Default {
                n191 = property on="Ring" class="Ring (strict)"("Visible"=FALSE) -> ()  [unwired: 2 in, 2 out]
                n192 = property on="Slider" class="Slide (strict)"("Visible"=FALSE) -> ()  [unwired: 2 in, 2 out]
              }
              frame "Brightness  **", "Color Level  **", "Compression  **", "FPS  **", "Sharpness  **" {
                n193 = call <vilib>:"NT Read Number.vi"("Name"=w318) -> ("Numeric"=w317:dbl)  [unwired: 9 in, 1 out]
                n194 = local write "Slider"(w317) -> ()
                n195 = property on="Slider" class="Slide (strict)"("Visible"=TRUE, "Scale.Maximum"=100.0 ("Scale.Range:Maximum")) -> ()  [unwired: 2 in, 2 out]
                n196 = property on="Ring" class="Ring (strict)"("Visible"=FALSE) -> ()  [unwired: 2 in, 2 out]
              }
            }
          }
        }
        n197 = property on="Progress" class="Clust (strict)"("Visible"=FALSE) -> ()  [unwired: 2 in, 2 out]
      }
      event "Test Name": Mouse Enter {
        # "Populate the ring with the list of tests"
        n198 = event-data() -> ()  [unwired: 1 in, 1 out]
        n199 = call <vilib>:"NT Read String Array.vi"("Name"="TestMode/TestList") -> ("String Array"=w325:string[])  [unwired: 9 in, 1 out]
        n200 = Build Array (concatenate)("Select the test to run...", w325) -> (w324:string[])
        n201 = property on="Test Name" class="Ring (strict)"("Strings []"=w324) -> ()  [unwired: 2 in, 2 out]
      }
      event "Test Name": Value Change {
        w327 = FALSE ("Visible")
        # "Tell the robot the test name to run"
        n202 = event-data() -> ("NewVal"=w331:u16)  [unwired: 1 in]
        n203 = property on="Test Name" class="Ring (strict)"() -> ("Strings []"=w332:string[])  [unwired: 2 in, 2 out]
        n204 = local write "Progress"(T6 {"Test Progress"=0, "Test Progress Text"=""} ("Progress")) -> ()
        n205 = Index Array(array=w332, index=w331) -> (element=w330:string)
        n206 = call <vilib>:"NT Write String.vi"("String"=w330, "Name"="TestMode/TestName") -> ()  [unwired: 9 in, 1 out]
        n207 = property on="Progress" class="Clust (strict)"("Visible"=TRUE) -> ()  [unwired: 2 in, 2 out]
        n208 = property on="Motor" class="Clust (strict)"("Visible"=w327) -> ()  [unwired: 2 in, 2 out]
        n209 = property on="Slider" class="Slide (strict)"("Visible"=w327) -> ()  [unwired: 2 in, 2 out]
        n210 = property on="On/Off" class="Bool (strict)"("Visible"=w327) -> ()  [unwired: 2 in, 2 out]
        n211 = property on="Rev/Fwd" class="Clust (strict)"("Visible"=w327) -> ()  [unwired: 2 in, 2 out]
        n212 = property on="Ring" class="Ring (strict)"("Visible"=w327) -> ()  [unwired: 2 in, 2 out]
      }
      event "Listbox": Double Click {
        n213 = event-data() -> ("PlatMods.Shift"=w335:bool, "Row"=w337:i32)  [unwired: 1 in]
        n214 = case shown="False" w335 {
          tunnel: w337 -> [w341 _]
          tunnel: 1 -> [w340 _]
          frame False {
            n215 = property on="Listbox" class="LstBox (strict)"() -> ("Item Symbols"=w339:i32[])  [unwired: 2 in, 2 out]
            n216 = Replace Array Subset(array=w339, new element=w340, index=w341) -> (w338:i32[])
            n217 = property on="Listbox" class="LstBox (strict)"("Item Symbols"=w338) -> ()  [unwired: 2 in, 2 out]
          }
          frame True {
            w342 = 0 ("Top Row")
            n218 = property on="Listbox" class="LstBox (strict)"() -> ("Number of Rows"=w344:u32)  [unwired: 2 in, 2 out]
            n219 = Initialize Array(0, w344) -> (w343:i32[])
            n220 = property on="Listbox" class="LstBox (strict)"("Top Row"=w342, "Value"=w342, "Item Symbols"=w343) -> ()  [unwired: 2 in, 2 out]
          }
        }
      }
      event "Listbox": Key Down {
        n221 = event-data() -> ("VKey"=w348:T13)  [unwired: 1 in]
        n222 = case shown="\"Left\", \"Right\"" w348 {
          selector: w348 -> [w353 _]
          tunnel: eventvkey."Left" ("VKey") -> [w351 _]
          frame "Left", "Right" {
            n223 = Equal?(x=w351, y=w353) -> (x = y?=w352:bool)
            n224 = Select(t=0, s=w352, f=1) -> (s? t:f=w354:i32)
            n225 = property on="Listbox" class="LstBox (strict)"() -> ("Item Symbols"=w357:i32[])  [unwired: 2 in, 2 out]
            n226 = Replace Array Subset(array=w357, new element=w354, index="Listbox") -> (w356:i32[])
            n227 = property on="Listbox" class="LstBox (strict)"("Item Symbols"=w356) -> ()  [unwired: 2 in, 2 out]
          }
          frame Default {
          }
        }
      }
      event "DB Camera Config": Value Change {
        n228 = event-data() -> ("NewVal"=w361:bool)  [unwired: 1 in]
        n229 = case shown="False" w361 {
          tunnel: w360 -> [w370 _]
          tunnel: [w363 w381] -> w359
          tunnel: w358 -> [w362 w381]
          frame False {
            w377 = "Camera"
            w380 = FALSE ("Visible")
            n230 = local read "Camera Settings"() -> (w369:T4)
            n231 = Index Array(array=w370) -> (element=w373:cluster{string[]})  [unwired: 1 in]
            n232 = Unbundle(w369) -> ("Frate Rate"=w368:i32, "Compression"=w367:i32, "Size"=w371:u16)
            n233 = Unbundle(w373) -> (w372:string[])
            n234 = Index Array(array=w372, index=w371) -> (element=w366:string)
            n235 = call-poly <vilib>:"Write Key.vi"("section"=w377, "value"=w366, "key"="Size", "refnum"=w362) -> ("refnum out"=w379:T12)  [unwired: 2 in, 5 out]
            n236 = call-poly <vilib>:"Write Key.vi"("section"=w377, "value"=w368, "key"="FrameRate", "refnum"=w379) -> ("refnum out"=w378:T12)  [unwired: 1 in, 6 out]
            n237 = property on="Camera Settings" class="Clust (strict)"("Visible"=w380) -> ()  [unwired: 2 in, 2 out]
            n238 = local write "DB Camera Config"(w380) -> ()
            n239 = call-poly <vilib>:"Write Key.vi"("section"=w377, "value"=w367, "key"="Compression", "refnum"=w378) -> ("refnum out"=w364:T12)  [unwired: 1 in, 6 out]
            n240 = call <vilib>:"Close Config Data.vi"("refnum"=w364) -> ("file path"=w365:path)  [unwired: 2 in, 8 out]
            n241 = call <vilib>:"Open Config Data.vi"("configuration file path"=w365) -> ("refnum"=w363:T12)  [unwired: 8 in, 2 out]
          }
          frame True {
            n242 = property on="Camera Settings" class="Clust (strict)"("Visible"=TRUE) -> ()  [unwired: 2 in, 2 out]
          }
        }
      }
      event "Camera Settings": Value Change {
        n243 = event-data() -> ("NewVal"=w394:T4)  [unwired: 1 in]
        n244 = Index Array(array=w390) -> (element=w389:cluster{string[]})  [unwired: 1 in]
        n245 = Unbundle(w394) -> ("Frate Rate"=w385:i32, "Compression"=w384:i32, "Size"=w387:u16)
        n246 = Unbundle(w389) -> (w388:string[])
        n247 = Index Array(array=w388, index=w387) -> (element=w386:string)
        n248 = Format Into String(format string="%s   %dfps   %d%%", w386, w385, w384) -> (resulting string=w391:string)  [unwired: 2 in, 1 out]
        n249 = Build Array(w391) -> (w392:string[])
        n250 = property on="DB Camera Config" class="Bool (strict)"("Strings [4]"=w392) -> ()  [unwired: 2 in, 2 out]
      }
      event "Motor.Enable": Value Change {
        n251 = event-data() -> ("NewVal"=w400:bool)  [unwired: 1 in]
        n252 = Unbundle("Motor") -> ("Value"=w399:dbl)  [unwired: 1 out]
        n253 = Select(t=w399, s=w400, f=0.0) -> (s? t:f=w397:dbl)
        n254 = call <vilib>:"NT Write Number.vi"("Numeric"=w397, "Name"=w396) -> ()  [unwired: 9 in, 1 out]
      }
      event "Slider": Value Change {
        n255 = event-data() -> ("NewVal"=w403:dbl)  [unwired: 1 in]
        n256 = call <vilib>:"NT Write Number.vi"("Numeric"=w403, "Name"=w404) -> ()  [unwired: 9 in, 1 out]
      }
      event "On/Off": Value Change {
        n257 = event-data() -> ("NewVal"=w408:bool)  [unwired: 1 in]
        n258 = Boolean To (0,1)(Boolean=w408) -> (0, 1=w407:i16)
        n259 = call <vilib>:"NT Write Number.vi"("Numeric"=w407, "Name"=w406) -> ()  [unwired: 9 in, 1 out]
      }
      event "Rev/Fwd": Value Change {
        n260 = event-data() -> ("NewVal.Forward"=w416:bool, "NewVal.Reverse"=w415:bool)  [unwired: 1 in]
        n261 = Boolean To (0,1)(Boolean=w416) -> (0, 1=w412:i16)
        n262 = Boolean To (0,1)(Boolean=w415) -> (0, 1=w414:i16)
        n263 = Negate(x=w414) -> (-x=w413:i16)
        n264 = Add(x=w412, y=w413) -> (x+y=w411:i16)
        n265 = call <vilib>:"NT Write Number.vi"("Numeric"=w411, "Name"=w410) -> ()  [unwired: 9 in, 1 out]
      }
      event "Ring": Value Change {
        n266 = event-data() -> ("NewVal"=w420:u16)  [unwired: 1 in]
        n267 = property on="Ring" class="Ring (strict)"() -> ("Strings []"=w421:string[])  [unwired: 2 in, 2 out]
        n268 = Index Array(array=w421, index=w420) -> (element=w419:string)
        n269 = call <vilib>:"NT Write String.vi"("String"=w419, "Name"=w418) -> ()  [unwired: 9 in, 1 out]
      }
    }
  }
  n270 = Index Array(array=w17) -> (element=w18:cluster{string[]})  [unwired: 1 in]
  n271 = Unbundle(w18) -> (w16:string[])
  n272 = Match First String(2:w16, 3:w15) -> (0:w14:i32)  [unwired: 1 out]
  n273 = Bundle("value"=w20, "value"=w19, "index"=w14) -> (w8:cluster{"value":i32, "value":i32, "index":i32})  [unwired: 1 out]
  n274 = while {
    stop <- FALSE stop-if-true
    n275 = Stop(stop? (T)="stop? (T)") -> ()
  }
  n276 = property on="On/Off" class="Bool (strict)"("Visible"=w31) -> ()  [unwired: 2 in, 2 out]
  n277 = property on="Motor" class="Clust (strict)"("Visible"=w31) -> ()  [unwired: 2 in, 2 out]
  n278 = property on="Progress" class="Clust (strict)"("Visible"=w31) -> ()  [unwired: 2 in, 2 out]
  n279 = property on="Ring" class="Ring (strict)"("Visible"=w31) -> ()  [unwired: 2 in, 2 out]
  n280 = property on="Camera Settings" class="Clust (strict)"("Val(Sgnl)"=w8) -> ()  [unwired: 2 in, 2 out]
  n281 = property on="Rev/Fwd" class="Clust (strict)"("Visible"=w31) -> ()  [unwired: 2 in, 2 out]
  n282 = property on="Camera Settings" class="Clust (strict)"("Visible"=w31) -> ()  [unwired: 2 in, 2 out]
  n283 = local write "DB Camera Config"(w31) -> ()
